vi "norm_vec_single.vi"(4 "vector":sgl[](array[numeric])) -> (0 "magnitude":sgl, 1 "normalized vector":sgl[](array[numeric]))   [LabVIEW 2013]
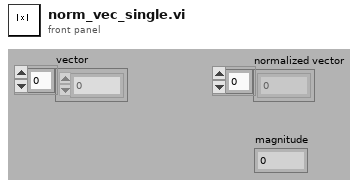
[diagram p1: front panel]
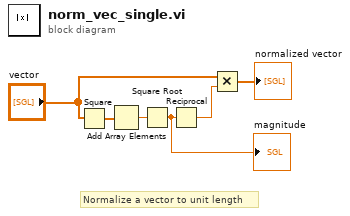
[diagram p0: block diagram]
diagram:
  # "Normalize a vector to unit length"
  n1 = Square(x="vector") -> (x^2=w6:sgl[])
  n2 = Add Array Elements(numeric array=w6) -> (sum=w5:sgl)
  n3 = Square Root(x=w5) -> (sqrt(x)=w1:sgl)
  "magnitude" <- w1
  n4 = Reciprocal(x=w1) -> (1/x=w4:sgl)
  n5 = Multiply ("Multiply.vi")(x="vector", y=w4) -> (x*y=→"normalized vector":sgl[])
